vi "Builder.Buffer.Parse.vi"(6 "VS Channel Buffer in":dbl[](array[numeric]), 7 "Data Type Buffers in":T5, 8 "error in (no error)":errorcluster, 10 "command":T3, 11 "Builder in":refnum<class "Builder.lvclass">) -> (0 "error out":errorcluster, 2 "response":T1, 3 "Builder out":refnum<class "Builder.lvclass">, 4 "VS Channel Buffer out":dbl[](array[numeric]), 5 "Data Type Buffers out":T5)   [LabVIEW 2016, in "DSF.Engine.lvlib" / "Builder.lvclass"]
uses:
  Builder.lvclass
  DSF.Engine.Typedefs.Type Buffers.ctl
  Interface/DSF.Engine.Interface.Builder.Command Data.ctl
  Interface/DSF.Engine.Interface.Builder.Command.ctl
  Interface/DSF.Engine.Interface.Builder.Response Data.ctl
  Interface/DSF.Engine.Interface.Builder.Response.ctl
  Builder.lvclass/Builder.ctl
  Cache/DSF.Engine.Memory.Cache.Plugin.lvclass/DSF.Engine.Memory.Cache.Plugin.ctl
  Cache/DSF.Engine.Memory.Cache.Transfer Group.lvclass/DSF.Engine.Memory.Cache.Transfer Group.ctl
  Cache/DSF.Engine.Memory.Cache.Transfer.lvclass/DSF.Engine.Memory.Cache.Transfer.ctl
  Shared/Classes/Transfer/DSF.Shared.Configuration.Transfer.lvclass/DSF.Shared.Configuration.Transfer.ctl
  Cache/DSF.Engine.Memory.Cache.Transfer Group.Get Transfer Caches.vi
  Cache/DSF.Engine.Memory.Cache.Plugin.Get Transfer Group Caches.vi
  Buffer/DSF.Engine.Memory.Buffer.lvclass
  Pointer/DSF.Engine.Memory.Pointer.VS Channels.lvclass
  Cache/DSF.Engine.Memory.Cache.Transfer Group.lvclass
  Cache/DSF.Engine.Memory.Cache.Framework.lvclass
  Cache/DSF.Engine.Memory.Cache.Plugin.lvclass
  Cache/DSF.Engine.Memory.Cache.Transfer.lvclass
  Shared/Classes/Transfer/DSF.Shared.Configuration.Transfer.lvclass
  Interface/DSF.Engine.Interface.Builder.lvclass
  DSF.Engine.lvlib
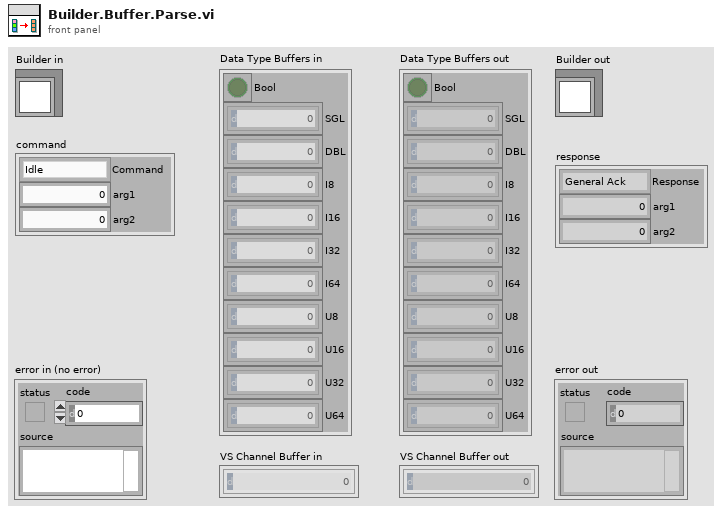
[diagram p1: front panel]
types:
  T1 = typedef "DSF.Engine.lvlib/DSF.Engine.Interface.Builder.lvclass/DSF.Engine.Interface.Builder.Response Data.ctl" = cluster{"Response":T2, "arg1":u64, "arg2":u64}
  T2 = typedef "DSF.Engine.lvlib/DSF.Engine.Interface.Builder.lvclass/DSF.Engine.Interface.Builder.Response.ctl" = enum8{"General Ack", "Initialize Complete", "Build Complete", "Parse Complete", "Shutdown Ack"}
  T3 = typedef "DSF.Engine.lvlib/DSF.Engine.Interface.Builder.lvclass/DSF.Engine.Interface.Builder.Command Data.ctl" = cluster{"Command":T4, "arg1":u64, "arg2":u64}
  T4 = typedef "DSF.Engine.lvlib/DSF.Engine.Interface.Builder.lvclass/DSF.Engine.Interface.Builder.Command.ctl" = enum8{"Idle", "Initialize", "Build Buffer", "Parse Buffer", "Shutdown"}
  T5 = typedef "DSF.Engine.lvlib/DSF.Engine.Typedefs.Type Buffers.ctl" = cluster{"Bool":bool[], "SGL":sgl[], "DBL":dbl[], "I8":i8[], "I16":i16[], "I32":i32[], "I64":i64[], "U8":u8[], "U16":u16[], "U32":u32[], "U64":u64[]}
  T6 = typedef "DSF.Engine.lvlib/Builder.lvclass/Builder.Command.Build-Parse.ctl" = cluster{"Command Byte":u8, "Plugin ID":i32, "Transfer Group ID":i32, "Transfer ID":i32, "unused":i32}
  T7 = typedef "DSF.Shared.lvlib/DSF.Shared.Typedefs.Configuration.Transfer.Channel Block Descriptor.ctl" = cluster{"First Channel Descriptor":T8, "count":u64, "vs channel index":u64}
  T8 = typedef "DSF.Shared.lvlib/DSF.Shared.Typedefs.Configuration.Transfer.Channel Descriptor.ctl" = cluster{"Channel Parameters":T9, "VS Channel Ref":T11}
  T9 = typedef "DSF.Shared.lvlib/DSF.Shared.Typedefs.Configuration.Transfer.Channel Parameters.ctl" = cluster{"offset":u64, "data type":T10}
  T10 = typedef "DSF.Shared.lvlib/DSF.Shared.Typedefs.Data Type.ctl" = enum8{"Bool", "SGL", "DBL", "I8", "I16", "I32", "I64", "U8", "U16", "U32", "U64"}
  T11 = typedef "Custom Device API.lvlib/Custom Device Item Ref.ctl" = u64
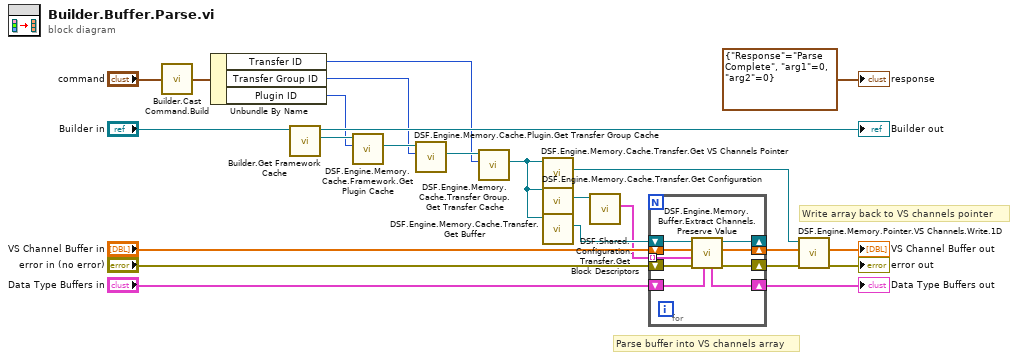
[diagram p0: block diagram]
diagram:
  # "Parse buffer into VS channels array"
  # "Write array back to VS channels pointer"
  n1 = call "Builder.Cast Command.Build.vi"("command"="command") -> ("build/parse command"=w2:T6)
  n2 = Unbundle By Name(w2) -> ("Transfer ID"=w14:i32, "Transfer Group ID"=w13:i32, "Plugin ID"=w15:i32)
  n3 = call "Builder.Get Framework Cache.vi"("Builder in"="Builder in") -> ("Framework Cache"=w19:refnum<class "DSF.Engine.Memory.Cache.Framework.lvclass">, "Builder out"=→"Builder out":refnum<class "Builder.lvclass">)  [unwired: 9 in]
  n4 = call "DSF.Engine.Memory.Cache.Framework.Get Plugin Cache.vi"("Plugin ID"=w15, "Framework Cache in"=w19) -> ("Plugin Cache"=w18:refnum<class "DSF.Engine.Memory.Cache.Plugin.lvclass">)  [unwired: 8 in, 1 out]
  n5 = call "DSF.Engine.Memory.Cache.Plugin.Get Transfer Group Cache.vi"("Transfer Group ID"=w13, "Plugin Cache in"=w18) -> ("Transfer Group Cache"=w17:refnum<class "DSF.Engine.Memory.Cache.Transfer Group.lvclass">)  [unwired: 8 in, 1 out]
  n6 = call "DSF.Engine.Memory.Cache.Transfer Group.Get Transfer Cache.vi"("Transfer ID"=w14, "Transfer Group Cache in"=w17) -> ("Transfer Cache"=w7:refnum<class "DSF.Engine.Memory.Cache.Transfer.lvclass">)  [unwired: 8 in, 1 out]
  n7 = call "DSF.Engine.Memory.Cache.Transfer.Get VS Channels Pointer.vi"("Transfer Cache in"=w7) -> ("VS Channels Pointer"=w6:refnum<class "DSF.Engine.Memory.Pointer.VS Channels.lvclass">)  [unwired: 9 in, 1 out]
  n8 = call "DSF.Engine.Memory.Cache.Transfer.Get Configuration.vi"("Transfer Cache in"=w7) -> ("Transfer Configuration"=w16:refnum<class "DSF.Shared.Configuration.Transfer.lvclass">)  [unwired: 9 in, 1 out]
  n9 = call "DSF.Engine.Memory.Cache.Transfer.Get Buffer.vi"("Transfer Cache in"=w7) -> ("Buffer"=w5:refnum<class "DSF.Engine.Memory.Buffer.lvclass">)  [unwired: 9 in, 1 out]
  n10 = call "DSF.Shared.Configuration.Transfer.Get Block Descriptors.vi"("Transfer Configuration in"=w16) -> ("Channel Blocks"=w4:T7[])  [unwired: 8 in, 2 out]
  n11 = for {
    shift-right: [w31] -> w23
    shift-left: "VS Channel Buffer in" -> [w32]
    shift-right: [w30] -> w20
    shift-left: "error in (no error)" -> [w33]
    shift-right: [w27] -> w21
    shift-left: "Data Type Buffers in" -> [w28]
    shift-right: [w26] -> _
    shift-left: w5 -> [w29]
    tunnel: w4 -> [w25] mode=indexing
    n12 = call "DSF.Engine.Memory.Buffer.Extract Channels.Preserve Value.vi"("Data Type Buffers in"=w28, "error in (no error)"=w33, "Channel Block"=w25, "VS Channels Array in"=w32, "Buffer in"=w29) -> ("error out"=w30:errorcluster, "VS Channels Array out"=w31:dbl[], "Buffer out"=w26:refnum<class "DSF.Engine.Memory.Buffer.lvclass">, "Data Type Buffers out"=w27:T5)  [unwired: 3 in]
  }
  "Data Type Buffers out" <- w21
  n13 = call "DSF.Engine.Memory.Pointer.VS Channels.Write.1D.vi"("error in (no error)"=w20, "Channels Array in"=w23, "VS Channels Pointer in"=w6) -> ("error out"=→"error out":errorcluster, "Channels Array out"=→"VS Channel Buffer out":dbl[])  [unwired: 5 in, 2 out]
  "response" <- T1 {"Response"=enum."Parse Complete", "arg1"=0, "arg2"=0} ("response")
